vi "SR430.set trigger slope.vi"(0 "i ref in":refnum<vi>, 2 "trigger slope":bool, 5 "error in (no error)":errorcluster) -> (14 "i ref out":refnum<vi>, 19 "error out":errorcluster)   [LabVIEW 2014, in "SR430.lvlib"]
doc: "Sets the trigger slope at the SR430. If the value is \"1\", the device triggers on the rising slope."
uses:
  SR430.lvlib
  CS_Core/CSSystem/CoreDefs/CoreDefs.error_type.ctl
  instr.lib/SR430/SR430Driver.lvlib
  CS_Core/CSSystem/CoreLib/CoreLib.lvlib
  CS_Core/CSApplicationBaseClasses/MCSBase/MCSBase.lvlib
  CSlibraries/UtilityLib/UtilityLib.lvlib
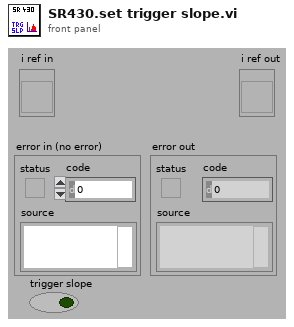
[diagram p1: front panel]
types:
  T1 = typedef "CoreDefs.error_type.ctl" = enum16{"no error", "can't load process", "can't unload process", "process does not exist", "can't install process", "can't remove process", "unknown function", "time out", "can't execute function", "duplicate queue name", "super not found", "caller queue invalid", "can't ping process", "unknown error", "VISA Error", "VISA timeout", "GPIB timeout", "GPIB error", "communication error", "data type mismatch", "can't read data from OPC server", "can't write data to OPC server", "OET error", "function not implemented", "process already exists", "invalid Shared Variable name", "error writing Shared Variable", "error reading Shared Variable", "invalid client name", "corrupt database", "unknown class", "call not authorized", "parameter out of range", "OET timeout: can't get data to modify", "invalid queue name", "requested operation incompatible with current state", "event undefined", "event disabled", "state undefined", "caller is not a friend", "EventBuilder: bad eventID", "EventBuilder: no DAQ devices", "a thread must not stop itself", "UNUSED ELEMENT4", "DiscArchiver: eventData incomplete", "DiscArchiver: eventData does not belong to run", "DiscArchiver: can't open file", "DiscArchiver: can't write to file", "DiscArchiver: available disc space low", "can't acquire semaphore", "error reading data from database", "notifier object is not existing", "can't register process", "can't unregister process", "illegal event type", "object disabled", "object already exists", "can't change state", "Instrument not found", "no connection to remote node", "invalid reference", "N/A", "UNUSED ELEMENT 1", "element not found", "illegal TCP/IP connection detected", "object does not exist", "invalid access ID", "unknown CS system", "invalid privilige", "unsupported data type", "unsupported server type", "IO server already exists", "Shared Variable already exists"}
  T2 = typedef "SR430Driver.lvlib/SR430_VISA Control.ctl" = cluster{"VISA resource name":refnum<visa-resource-name>}
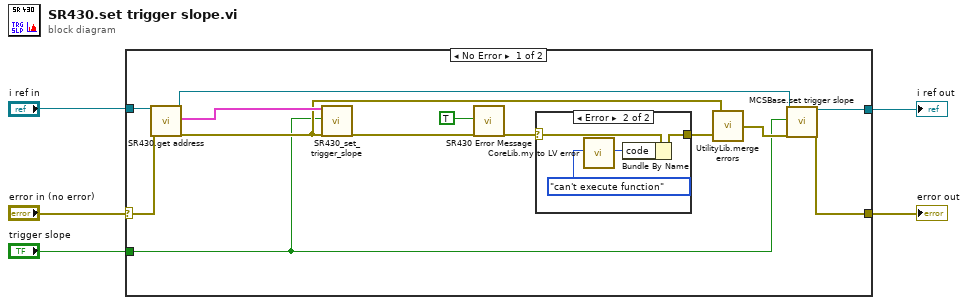
[diagram p0: block diagram]
diagram:
  n1 = case shown="No Error" "error in (no error)" {
    selector: "error in (no error)" -> [w11 w24]
    tunnel: "i ref in" -> [w18 w25]
    tunnel: "trigger slope" -> [w6 _]
    tunnel: [w7 w24] -> w3
    tunnel: [w8 w25] -> w2
    frame No Error {
      n2 = call "SR430.get address.vi"("i ref in"=w18, "error in (no error)"=w11) -> ("i ref out"=w9:refnum<vi>, "address"=w17:T2, "error out"=w16:errorcluster)  [unwired: 15 in]
      n3 = call "SR430_set_trigger_slope.vi"("address"=w17, "triggerSlope"=w6, "error in (no error)"=w16) -> ("error out"=w12:errorcluster)  [unwired: 15 in, 1 out]
      n4 = call "SR430 Error Message.vi"("addMessageToSource"=TRUE ("add message to source"), "error in (no error)"=w12) -> ("error out"=w15:errorcluster)  [unwired: 14 in, 3 out]
      n5 = case shown="Error" w15 {
        selector: w15 -> [w19 w23]
        tunnel: [w19 w20] -> w13
        frame No Error {
        }
        frame Error {
          n6 = call "CoreLib.my to LV error.vi"("ErrorTypes"=CoreDefs.error_type."can't execute function") -> ("LV error code"=w22:i32)  [unwired: 17 in, 1 out]
          n7 = Bundle By Name(cluster=w23, "code"=w22) -> (w20:errorcluster)
        }
      }
      n8 = call "UtilityLib.merge errors.vi"("error2 (no error)"=w13, "error1 (no error)"=w16) -> ("error out"=w10:errorcluster)
      n9 = call "MCSBase.set trigger slope.vi"("i ref in"=w9, "triggerSlope"=w6, "error in (no error)"=w10) -> ("i ref out"=w8:refnum<vi>, "error out"=w7:errorcluster)  [unwired: 14 in, 1 out]
    }
    frame Error {
    }
  }
  "error out" <- w3
  "i ref out" <- w2
